vi "Read OldLibPath.vi"(11 "ProjectItem in":refnum<class "Search.lvclass">) -> (2 "OldLibPath":path, 3 "ProjectItem out":refnum<class "Search.lvclass">)   [LabVIEW 2016, in "Search.lvclass"]
uses:
  Search.lvclass
  Search.lvclass/Search.ctl
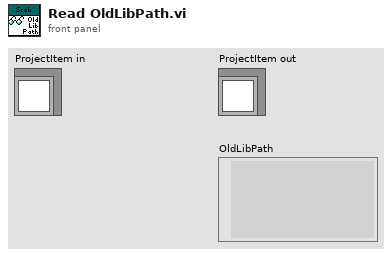
[diagram p1: front panel]
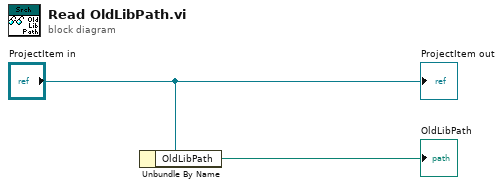
[diagram p0: block diagram]
diagram:
  n1 = Unbundle By Name("ProjectItem in") -> ("OldLibPath"=→"OldLibPath":path)
  "ProjectItem out" <- "ProjectItem in"
